vi "UI.vi"(0 "reference in":refnum<class "GUI Alarm Setting.lvclass">, 5 "error in (no error)":errorcluster) -> (14 "reference out":refnum<class "GUI Alarm Setting.lvclass">, 19 "error out":errorcluster)   [LabVIEW 2019, in "GUI Alarm Setting.lvclass"]
uses:
  GUI Alarm Setting.lvclass
  D:/GIT H4000/H4000/src/GUI_class/GUI.lvclass
  GUI_class/GUI.lvclass/GUI.ctl
  GUI_class/Set Win State.vi
  GUI_class/protected/GetSheredData.vi
  GUI_class/GUI.lvclass
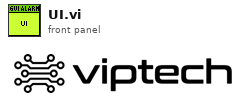
[diagram p1: front panel]
types:
  T1 = enum32{"Invalid", "Standard", "Closed", "Hidden", "Minimized", "Maximized"}
  T2 = enum32{"invalid app kind", "Development System", "Run Time System", "Student Edition", "Embedded LabVIEW", "Evaluation", "Custom"}
  T3 = cluster{"Core":cluster{"Current VI Reference":refnum<vi>, "Close Panel on Exit?":bool}, "file customer":string, "file developer":string, "valid data":bool}
  T4 = cluster{"Current VI Reference":refnum<vi>, "Close Panel on Exit?":bool}
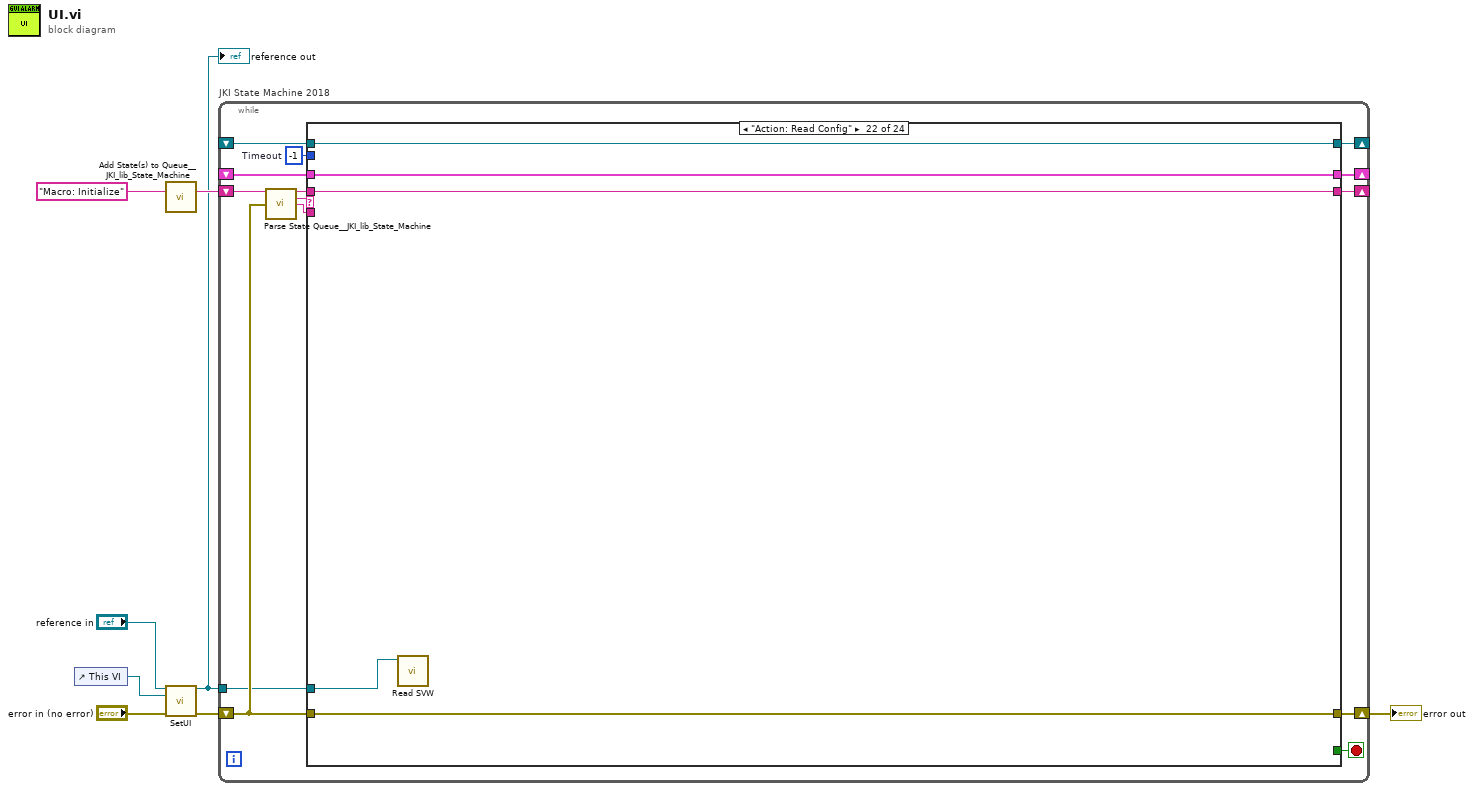
[diagram p0: block diagram]
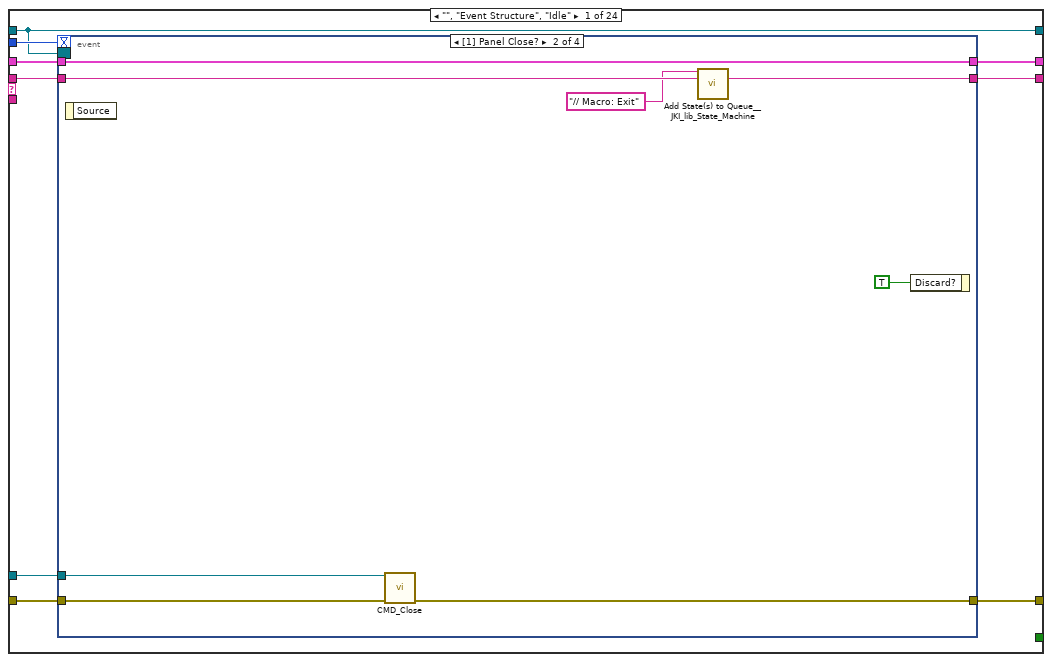
[diagram p2: hidden frame]
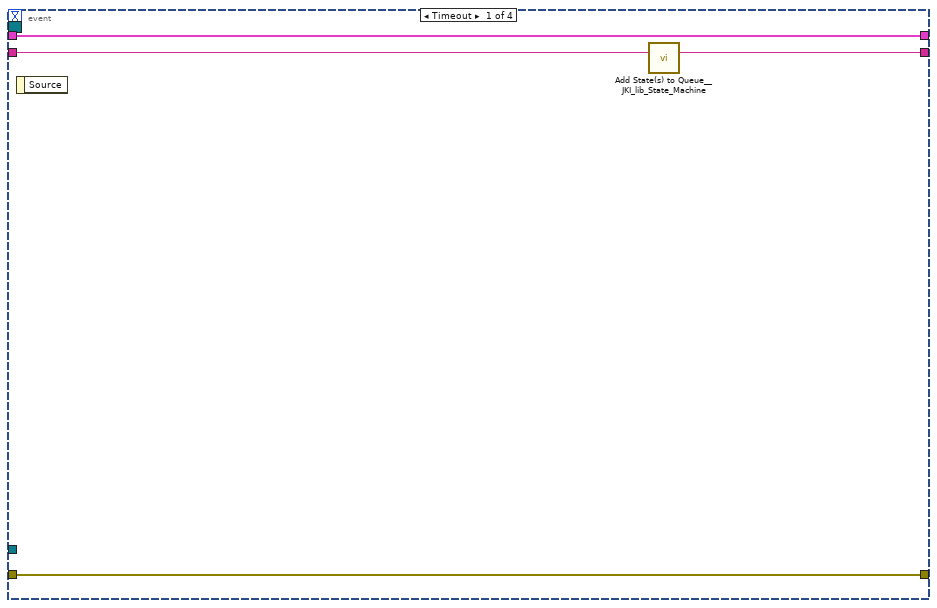
[diagram p3: hidden frame]
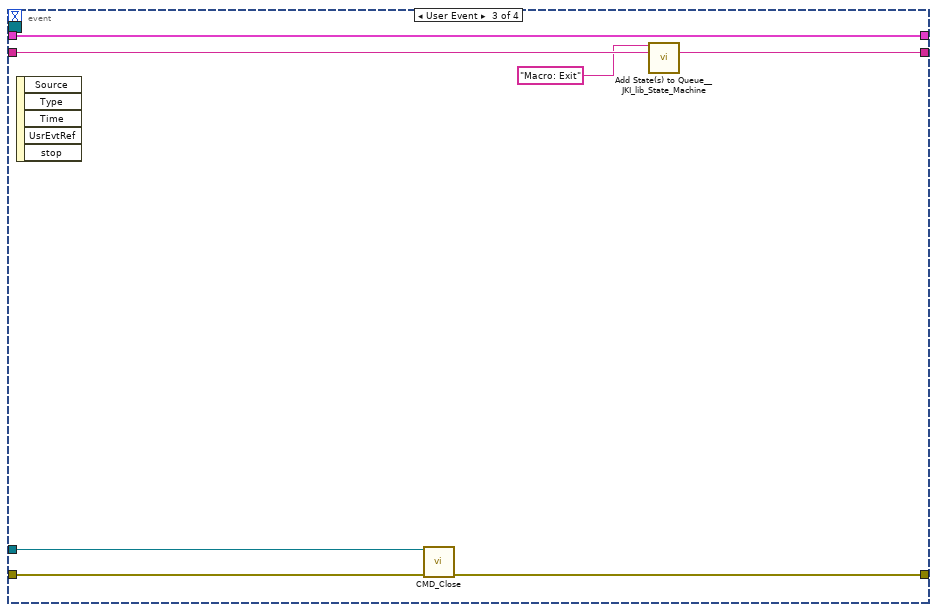
[diagram p4: hidden frame]
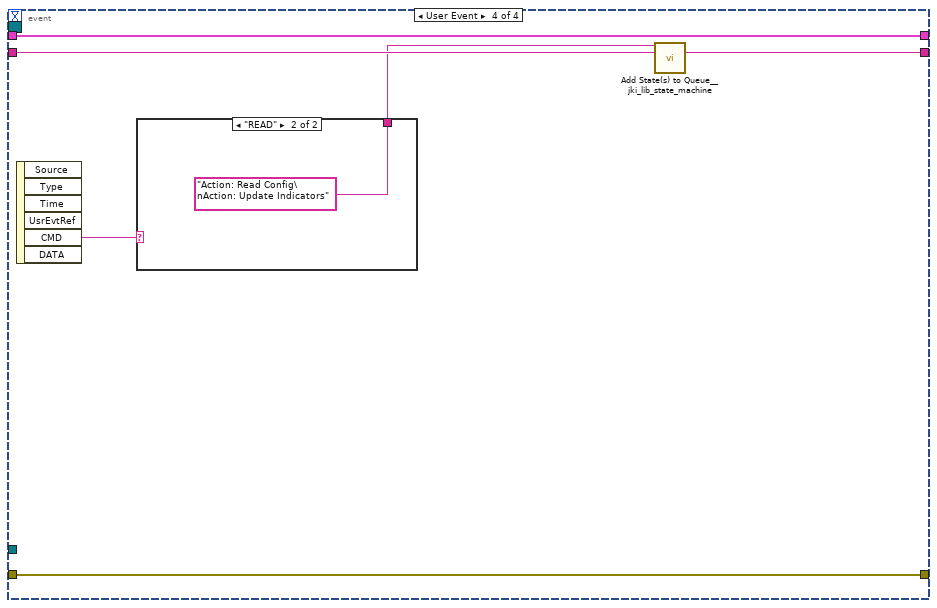
[diagram p5: hidden frame]
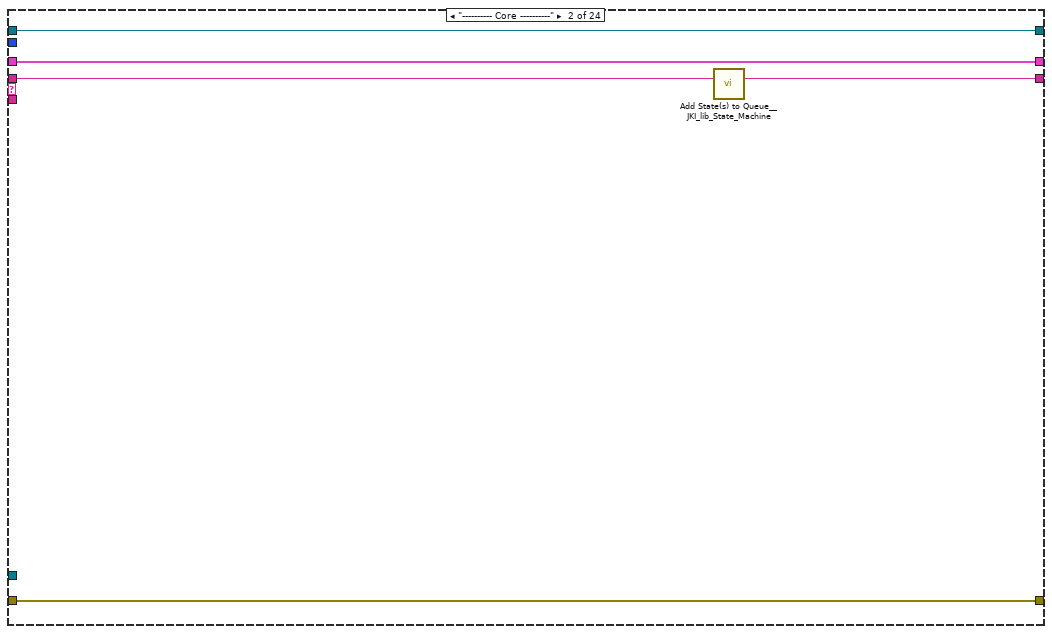
[diagram p7: hidden frame]
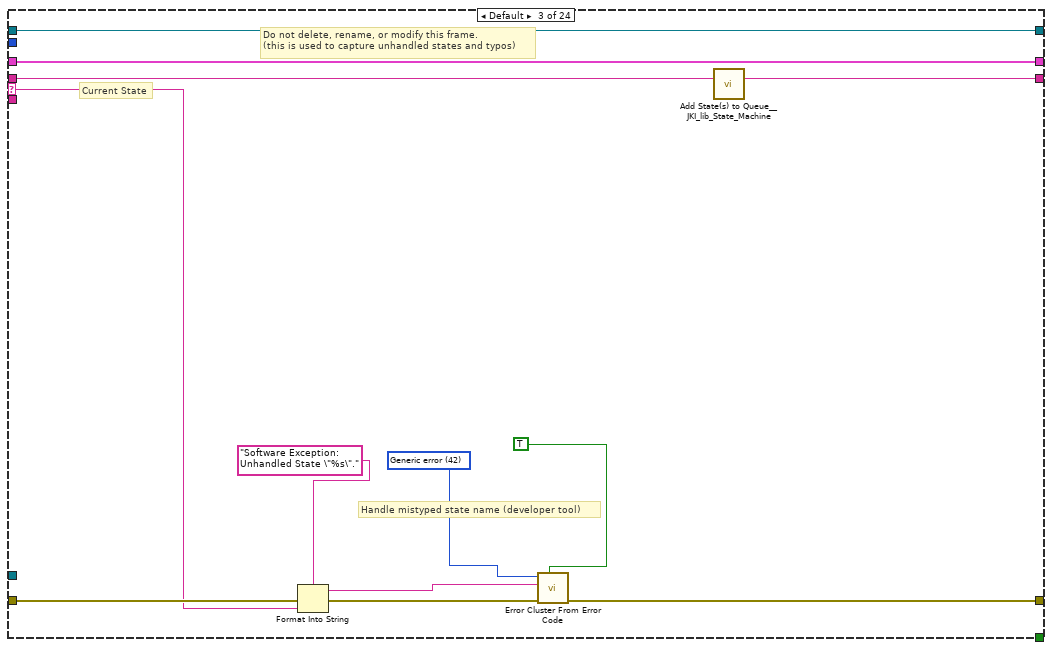
[diagram p8: hidden frame]
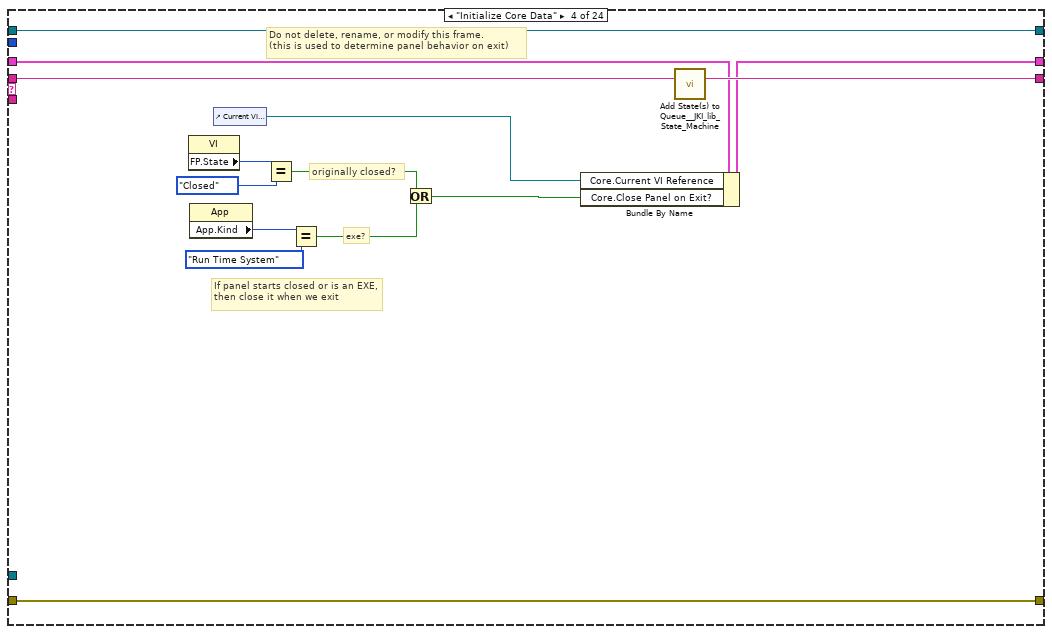
[diagram p9: hidden frame]
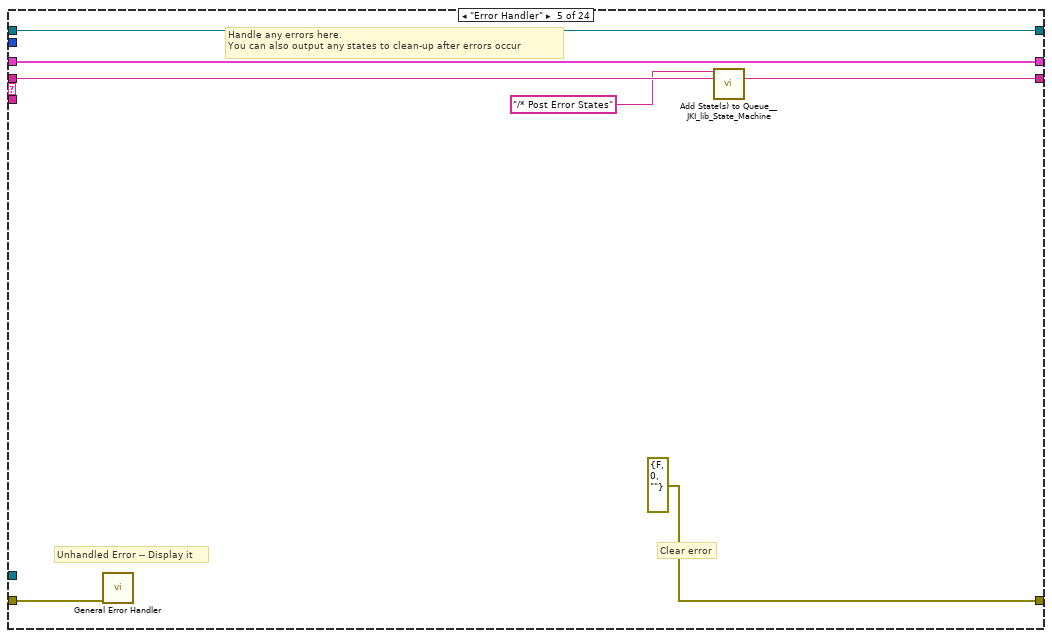
[diagram p10: hidden frame]
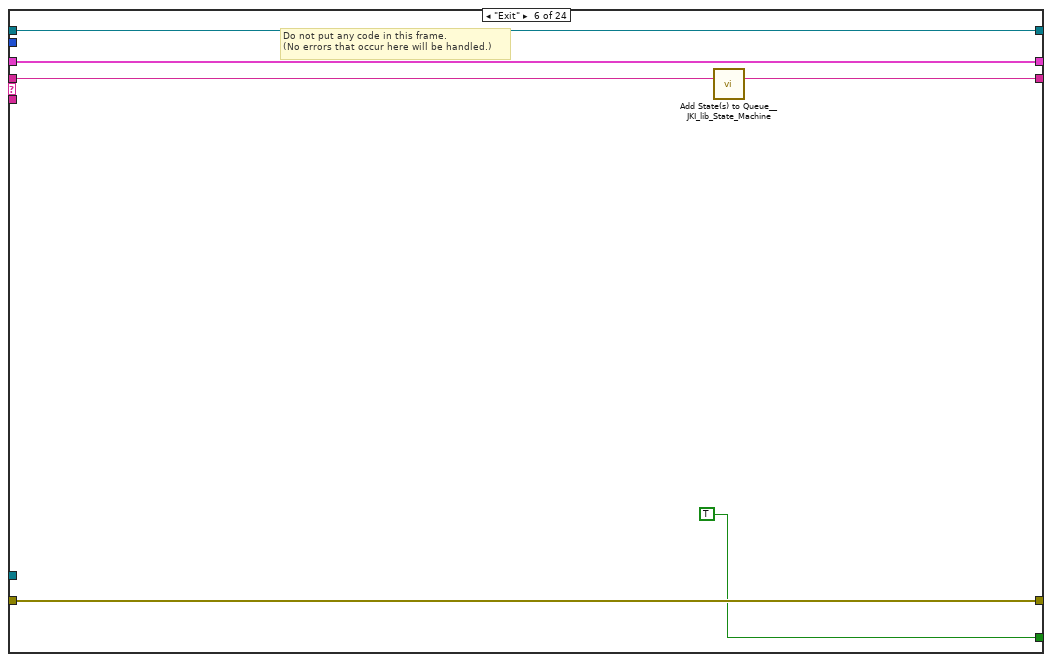
[diagram p11: hidden frame]
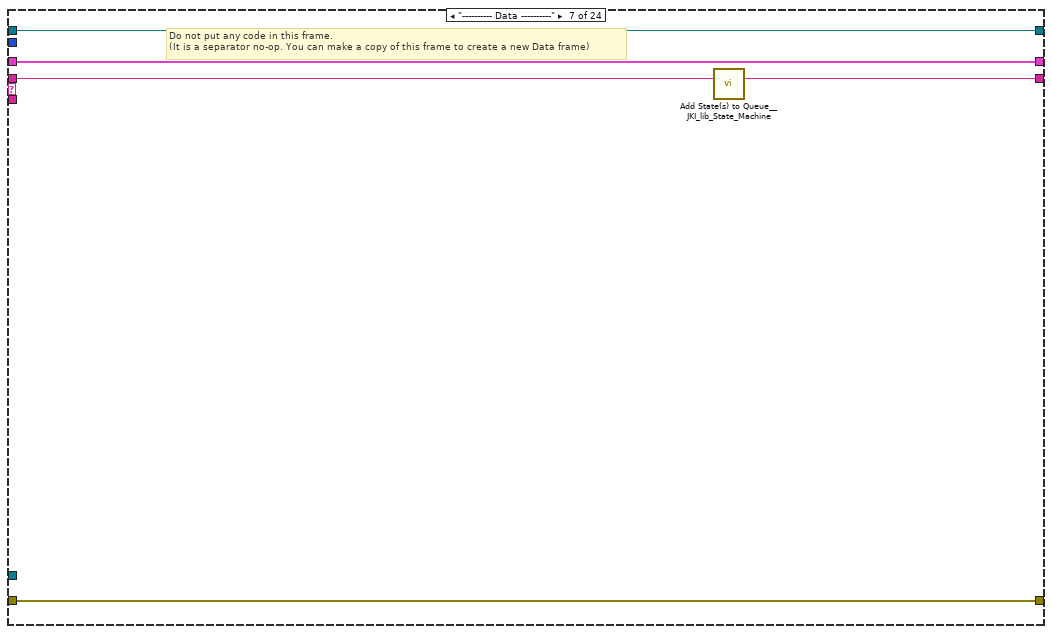
[diagram p12: hidden frame]
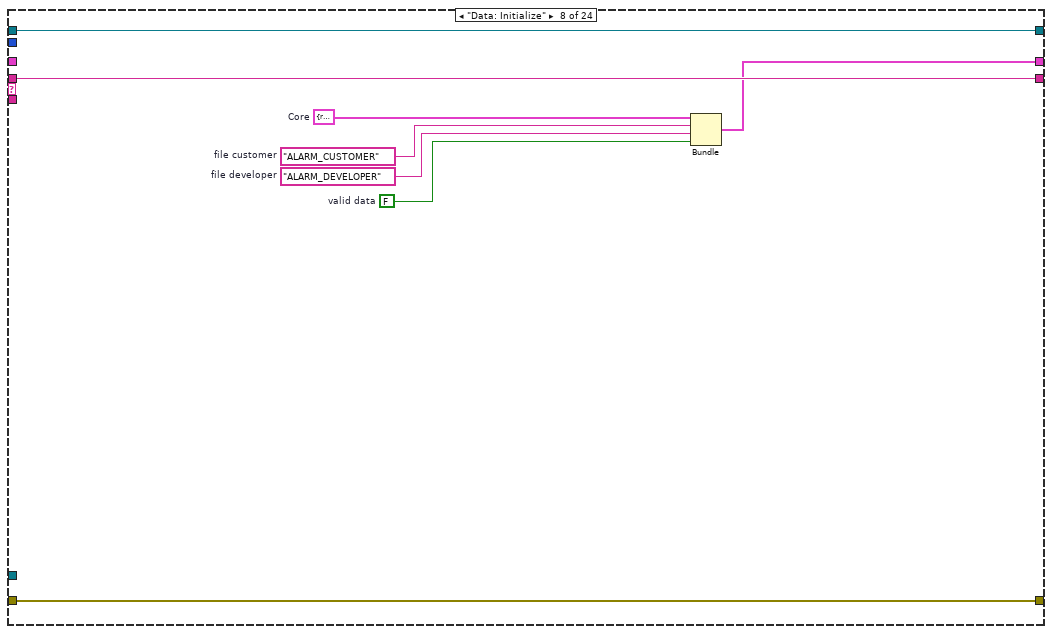
[diagram p13: hidden frame]
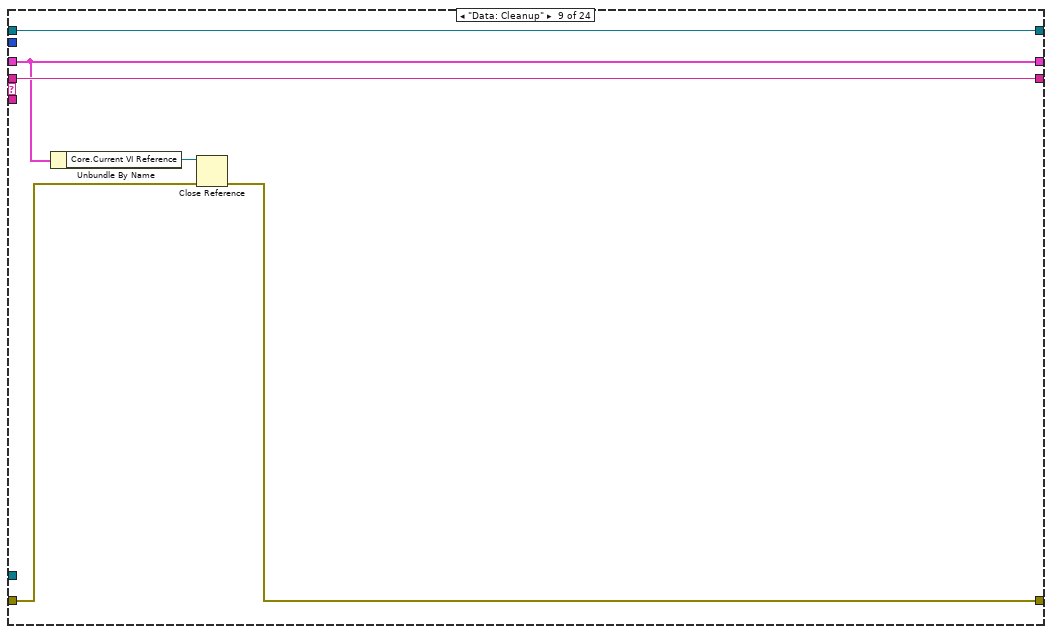
[diagram p14: hidden frame]
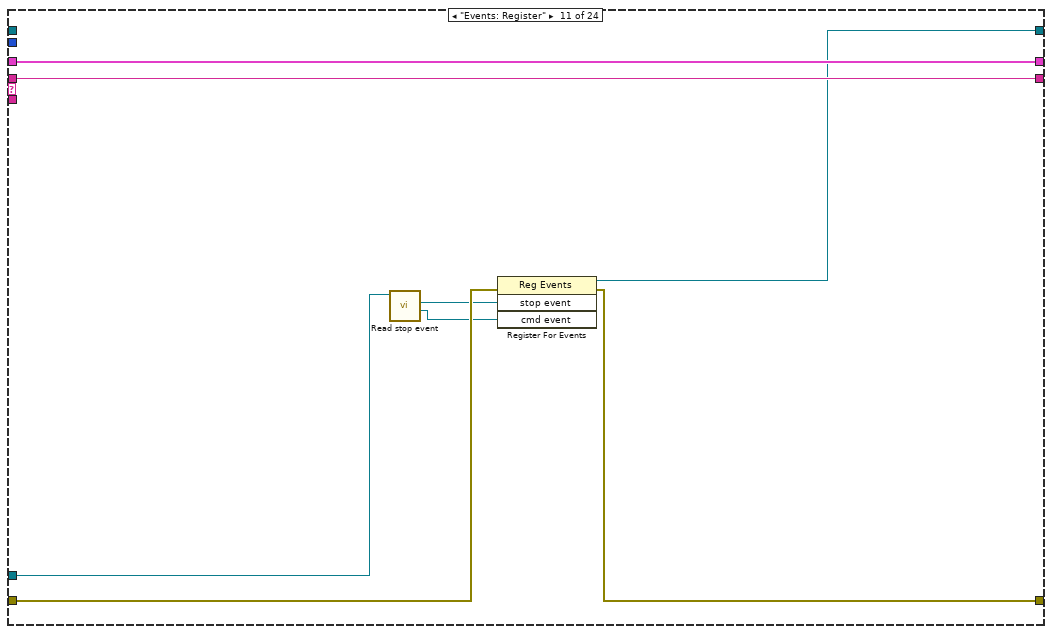
[diagram p16: hidden frame]
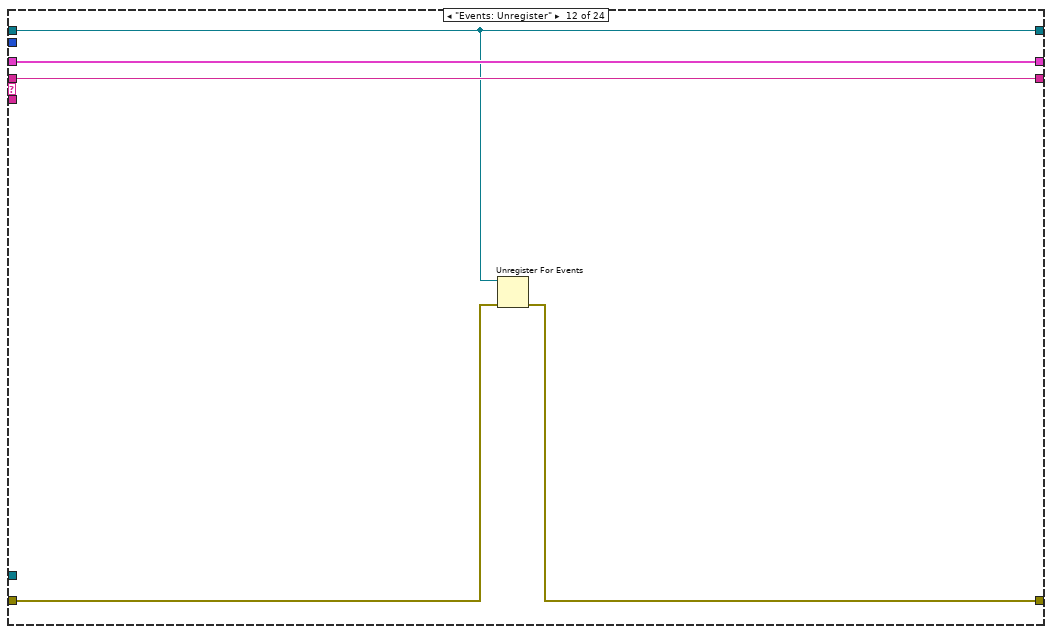
[diagram p17: hidden frame]
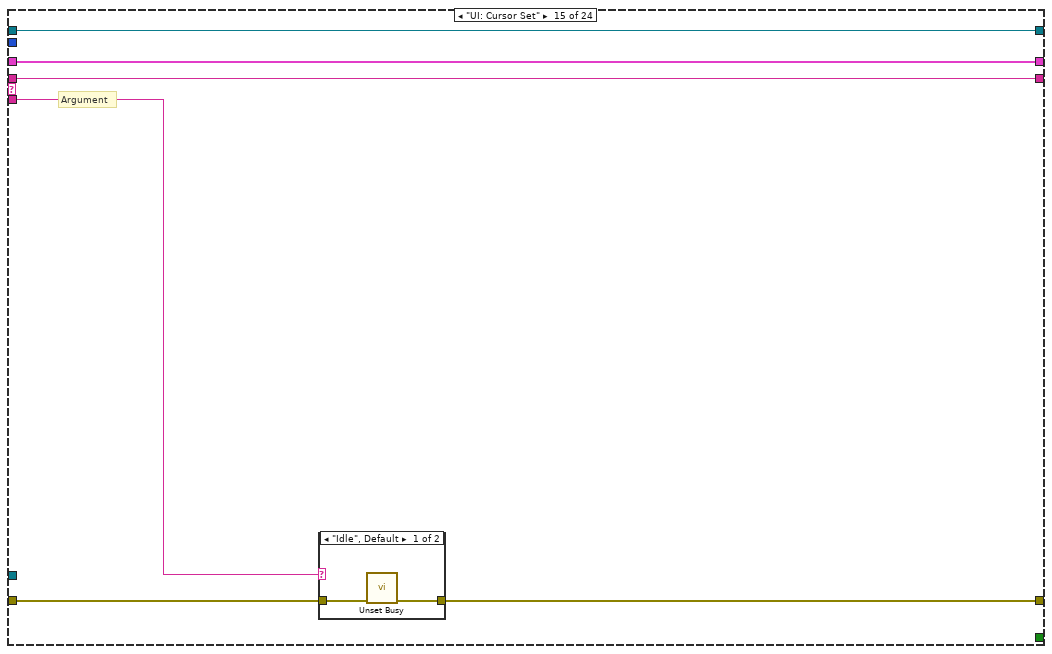
[diagram p20: hidden frame]
diagram:
  n1 = control-ref of="This VI"() -> (w3:refnum<vi>)
  n2 = call <vilib>:"Add State(s) to Queue__JKI_lib_State_Machine.vi"("State(s) in (\"\")"="Macro: Initialize") -> ("States Out"=w8:string)  [unwired: 14 in]
  n3 = call "SetUI.vi"("reference in"="reference in", "UI VI"=w3, "error in (no error)"="error in (no error)") -> ("reference out"=w1:refnum<class "GUI Alarm Setting.lvclass">, "error out"=w2:errorcluster)  [unwired: 11 in]
  "reference out" <- w1
  n4 = while "JKI State Machine 2018" {
    shift-right: [w15] -> _
    shift-left: _ -> [w14]
    shift-right: [w18] -> w6
    shift-left: w2 -> [w12]
    shift-right: [w17] -> _
    shift-left: w8 -> [w19]
    tunnel: w1 -> [w11]
    shift-right: [w10] -> _
    shift-left: _ -> [w9]
    stop <- w16 stop-if-true
    w13 = -1  # Timeout
    n5 = call <vilib>:"Parse State Queue__JKI_lib_State_Machine.vi"("State Queue"=w19, "Error In (no error)"=w12) -> ("Remaining States"=w21:string, "Current State"=w22:string, "Arguments"=w20:string)  [unwired: 11 in]
    n6 = case shown="\"Action: Read Config\"" w22 {
      selector: w22 -> [_ _ w64 _ _ _ _ _ _ _ _ _ _ _ _ _ _ _ _ _ _ _ _ _]
      tunnel: w21 -> [w31 w62 w68 w88 w95 w101 w106 w114 w120 w124 w132 w137 w141 w145 w151 w162 w231 w237 w243 w255 w259 w263 w268 w272]
      tunnel: w20 -> [_ _ _ _ _ _ _ _ _ _ _ _ _ _ w147 w157 _ _ _ _ _ _ _ _]
      tunnel: w14 -> [w29 w59 w66 w81 w92 w99 w103 _ w116 w122 w131 w136 w139 w144 w150 w159 w229 w234 w240 w252 w257 w260 w266 w269]
      tunnel: [w28 w60 w70 w85 errorcluster {"status"=FALSE, "code"=0, "source"=""} ("error out") w98 w104 w112 w117 w123 w129 w133 w140 w143 w148 w160 w230 w235 w241 w253 w258 w261 w265 w270] -> w18
      tunnel: w12 -> [w27 w60 w69 w85 w91 w98 w104 w112 w118 w123 w128 w134 w140 w143 w149 w161 w230 w235 w241 w253 w258 w261 w265 w270]
      tunnel: [w30 w61 w67 w87 w94 w100 w105 w114 w120 w124 w132 w137 w141 w145 w151 w162 w231 w236 w242 w254 w259 w263 w268 w272] -> w17
      tunnel: [_ _ _ _ _ TRUE _ _ _ _ _ _ _ _ _ _ _ _ _ _ _ _ _ _] -> w16
      tunnel: [w26 w59 w66 w86 w92 w99 w103 w113 w116 w122 w131 w136 w139 w144 w150 w159 w229 w234 w240 w252 w257 w260 w266 w269] -> w15
      tunnel: w13 -> [w25 _ _ _ _ _ _ _ _ _ _ _ _ _ _ _ _ _ _ _ _ _ _ _]
      tunnel: w11 -> [w24 _ _ _ _ _ _ _ _ _ w127 _ _ _ _ _ _ _ _ _ _ w262 _ _]
      tunnel: [w23 w58 w63 w75 w89 w96 w102 w110 w115 w121 w130 w135 w138 w142 w146 w156 w228 w232 w238 w245 w256 w264 w267 w271] -> w10
      tunnel: w9 -> [w23 w58 w63 w75 w89 w96 w102 w110 w115 w121 _ w135 w138 w142 w146 w156 w228 w232 w238 w245 w256 w264 w267 w271]
      frame "", "Event Structure", "Idle" {
        n7 = event shown="[1] Panel Close?" {
          selector: w23 -> [_ _ _ _]
          dyn-events: _ -> [_ _ _ _]
          timeout: w25 -> [_ _ _ _]
          tunnel: w31 -> [w35 w43 w50 w52]
          tunnel: [w34 w42 w49 w53] -> w30
          tunnel: w29 -> [w32 w41 w48 w55]
          tunnel: [w33 w36 w44 w56] -> w28
          tunnel: w27 -> [w33 w37 w45 w56]
          tunnel: [w32 w41 w48 w55] -> w26
          tunnel: w24 -> [_ w38 w46 _]
          event Timeout {
            n8 = event-data() -> ()  [unwired: 1 in, 1 out]
            n9 = call <vilib>:"Add State(s) to Queue__JKI_lib_State_Machine.vi"("State(s) in (\"\")"=w35) -> ("States Out"=w34:string)  [unwired: 14 in]
          }
          event Panel Close? {
            n10 = event-data() -> ()  [unwired: 1 in, 1 out]
            n11 = call "CMD_Close.vi"("reference in"=w38, "error in (no error)"=w37) -> ("error out"=w36:errorcluster)  [unwired: 12 in, 1 out]
            n12 = call <vilib>:"Add State(s) to Queue__JKI_lib_State_Machine.vi"("State(s) in Front (\"\")"="// Macro: Exit", "State(s) in (\"\")"=w43) -> ("States Out"=w42:string)  [unwired: 13 in]
            n13 = event-data("Discard?"=TRUE) -> ()  [unwired: 1 in, 1 out]
          }
          event User Event {
            n14 = event-data() -> ()  [unwired: 1 in, 5 out]
            n15 = call "CMD_Close.vi"("reference in"=w46, "error in (no error)"=w45) -> ("error out"=w44:errorcluster)  [unwired: 12 in, 1 out]
            n16 = call <vilib>:"Add State(s) to Queue__JKI_lib_State_Machine.vi"("State(s) in Front (\"\")"="Macro: Exit", "State(s) in (\"\")"=w50) -> ("States Out"=w49:string)  [unwired: 13 in]
          }
          event User Event {
            n17 = event-data() -> ("CMD"=w54:string)  [unwired: 1 in, 5 out]
            n18 = case shown="\"READ\"" w54 {
              tunnel: [_ "Action: Read Config\nAction: Update Indicators" ("State(s) in Front (\"\")")] -> w51
              frame "False", Default {
              }
              frame "READ" {
              }
            }
            n19 = call <vilib>:"Add State(s) to Queue__jki_lib_state_machine.vi"("State(s) in Front (\"\")"=w51, "State(s) in (\"\")"=w52) -> ("States Out"=w53:string)  [unwired: 13 in]
          }
        }
      }
      frame "---------- Core ----------" {
        n20 = call <vilib>:"Add State(s) to Queue__JKI_lib_State_Machine.vi"("State(s) in (\"\")"=w62) -> ("States Out"=w61:string)  [unwired: 14 in]
      }
      frame Default {
        w73 = 42 items=["No error", "Argument error", "Memory is full", "Out of zone", "End of file", "File already open", "Generic file I/O error", "File not found", "File permission error", "Disk is full", "Duplicate path", "Too many files open", "System feature not enabled", "Resource file not found", "Cannot add resource", "Resource not found", "Image not found", "Image memory error", "Pen does not exist", "Config type invalid", "Config token not found", "Config parse error", "Config memory error", "Bad external code format", "Bad external code offset", "External code not present", "Null window", "Destroy window error", "Null menu", "Print aborted", "Bad print record", "Print driver error", "Windows error during printing", "Memory error during printing", "Print dialog error", "Generic print error", "Invalid device refnum", "Device not found", "Device parameter error", "Device unit error", "Cannot open device", "Device call aborted", "Generic error", "Cancelled by user", "Object ID too low", "Object ID too high", "Object not in heap", "Unknown heap", "Unknown object (invalid DefProc)", "Unknown object (DefProc not in table)", "Message out of range", "Invalid (null) method", "Unknown message", "Manager call not supported", "Bad address", "Network operation in progress", "Network operation timed out", "Connection is busy", "Network attribute not supported", "Network error", "Address in use", "System out of memory", "Connection aborted", "Connection refused", "Not connected", "Already connected", "Connection closed", "Initialization error (interapplication manager)", "Bad occurrence", "Wait on unbound occurrence handler", "Occurrence queue overflow", "Datalog type conflict", "Unused", "Unrecognized type (interapplication manager)", "Memory corrupt", "Failed to make temporary DLL", "Old CIN version", "Drag socket not found", "Failed to load drop-object", "Failed to register OLE object", "Failed to release OLE object", "Format specifier type mismatch", "Unknown format specifier", "Too few format specifiers", "Too many format specifiers", "Scan failed", "Newer CIN version", "Error converting to variant", "Runtime menu error", "Password tampered", "Variant attribute not found", "Incompatible variant data type", "Event data is not available", "Event Store is not present", "Occurrence is not found", "Event Queue is not created", "Event info is not available", "Refnum passed is NULL", "Error retrieving Class GUID", "Error retrieving CoClass GUID", "Error retrieving TypeLib GUID.", "Bad built application magic bytes.", "Specific driver is different from the specific driver associated with the Logical Name.", "There is no session opened to the class driver.", "Max Error", "MAX - Error with config objects", "MAX - Error loading configuration", "MAX - Group not supported"]
        # "Current State"
        # "Do not delete, rename, or modify this frame.\n(this is used to capture unhandled states and typos)"
        # "Handle mistyped state name (developer tool)"
        n21 = Format Into String(format string="Software Exception: Unhandled State \"%s\"." ("message"), error in=w69, w64) -> (resulting string=w72:string, error out=w71:errorcluster)  [unwired: 1 in]
        n22 = call <vilib>:"Error Cluster From Error Code.vi"("show call chain? (False)"=TRUE, "error in (no error)"=w71, "error message (\"\")"=w72, "error code (0)"=w73) -> ("error out"=w70:errorcluster)  [unwired: 5 in]
        n23 = call <vilib>:"Add State(s) to Queue__JKI_lib_State_Machine.vi"("State(s) in (\"\")"=w68) -> ("States Out"=w67:string)  [unwired: 14 in]
      }
      frame "Initialize Core Data" {
        # "Do not delete, rename, or modify this frame.\n(this is used to determine panel behavior on exit)"
        # "originally closed?"
        # "exe?"
        # "If panel starts closed or is an EXE, then close it when we exit"
        n24 = property class="VI"() -> ("FP.State"=w78:T1)  [unwired: 2 in, 2 out]
        n25 = property class="App"() -> ("App.Kind"=w84:T2)  [unwired: 2 in, 2 out]
        n26 = control-ref of="Current VI Reference"() -> (w79:refnum<vi>)
        n27 = Equal?(x=w78, y=T1."Closed" ("Front Panel Window:State")) -> (x = y?=w76:bool)
        n28 = Equal?(x=w84, y=T2."Run Time System" ("Application:Kind")) -> (x = y?=w82:bool)
        n29 = Or(x=w76, y=w82) -> (x .or. y?=w80:bool)
        n30 = Bundle By Name(cluster=w81, "Core.Current VI Reference"=w79, "Core.Close Panel on Exit?"=w80) -> (w86:T3)
        n31 = call <vilib>:"Add State(s) to Queue__JKI_lib_State_Machine.vi"("State(s) in (\"\")"=w88) -> ("States Out"=w87:string)  [unwired: 14 in]
      }
      frame "Error Handler" {
        # "Unhandled Error -- Display it"
        # "Handle any errors here.\nYou can also output any states to clean-up after errors occur"
        # "Clear error"
        n32 = call <vilib>:"General Error Handler.vi"("error in (no error)"=w91) -> ()  [unwired: 10 in, 5 out]
        n33 = call <vilib>:"Add State(s) to Queue__JKI_lib_State_Machine.vi"("State(s) in Front (\"\")"="/* Post Error States", "State(s) in (\"\")"=w95) -> ("States Out"=w94:string)  [unwired: 13 in]
      }
      frame "Exit" {
        # "Do not put any code in this frame.\n(No errors that occur here will be handled.)"
        n34 = call <vilib>:"Add State(s) to Queue__JKI_lib_State_Machine.vi"("State(s) in (\"\")"=w101) -> ("States Out"=w100:string)  [unwired: 14 in]
      }
      frame "---------- Data ----------" {
        # "Do not put any code in this frame.\n(It is a separator no-op. You can make a copy of this frame to create a new Data frame)"
        n35 = call <vilib>:"Add State(s) to Queue__JKI_lib_State_Machine.vi"("State(s) in (\"\")"=w106) -> ("States Out"=w105:string)  [unwired: 14 in]
      }
      frame "Data: Initialize" {
        w107 = FALSE  # valid data
        w108 = "ALARM_DEVELOPER"  # file developer
        w109 = "ALARM_CUSTOMER"  # file customer
        w111 = T4 {"Current VI Reference"=refnum, "Close Panel on Exit?"=FALSE}  # Core
        n36 = Bundle("Core"=w111, "file customer"=w109, "file developer"=w108, "valid data"=w107) -> (w113:T3)  [unwired: 1 in]
      }
      frame "Data: Cleanup" {
        n37 = Unbundle By Name(w116) -> ("Core.Current VI Reference"=w119:refnum<vi>)
        n38 = Close Reference(reference=w119, error in (no error)=w118) -> (error out=w117:errorcluster)
      }
      frame "---------- Events ----------" {
      }
      frame "Events: Register" {
        n39 = call "Read stop event.vi"("GUI in"=w127) -> ("cmd event"=w125:refnum<user-event>, "stop event"=w126:refnum<user-event>)  [unwired: 8 in, 1 out]
        n40 = register-events(error in=w128, w126, w125) -> (reference out=w130:refnum<event-registration>, error out=w129:errorcluster)  [unwired: 1 in]
      }
      frame "Events: Unregister" {
        n41 = Unregister For Events(event registration refnum=w135, error in=w134) -> (error out=w133:errorcluster)
      }
      frame "---------- UI ----------" {
      }
      frame "UI: Initialize" {
      }
      frame "UI: Cursor Set" {
        # "Argument"
        n42 = case shown="\"Idle\", Default" w147 {
          tunnel: w149 -> [w153 w155]
          tunnel: [w152 w154] -> w148
          frame "Idle", Default {
            n43 = call <vilib>:"Unset Busy.vi"("error in (no error)"=w153) -> ("error out"=w152:errorcluster)  [unwired: 10 in]
          }
          frame "Busy" {
            n44 = call <vilib>:"Set Busy.vi"("error in (no error)"=w155) -> ("error out"=w154:errorcluster)  [unwired: 9 in, 1 out]
          }
        }
      }
      frame "UI: Front Panel State" {
        # "Argument"
        n45 = Unbundle By Name(w159) -> ("Core.Current VI Reference"=w158:refnum<vi>)
        n46 = case shown="\"Minimize\", \"Minimized\"" w157 {
          tunnel: w161 -> [w168 w183 w194 w207 w220]
          tunnel: [w170 w184 w196 w209 w222] -> w160
          tunnel: w158 -> [w169 w181 w195 w208 w221]
          frame "Open", "Standard", Default {
            w163 = T1."Standard" ("State")
            n47 = property class="VI"(reference=w169, error in=w168) -> (reference out=w166:refnum<vi>, error out=w167:errorcluster, "FP.State"=w165:T1)
            n48 = Not Equal?(x=w165, y=w163) -> (x != y?=w164:bool)
            n49 = case shown="True" w164 {
              tunnel: [w174 w176] -> w170
              tunnel: w167 -> [w173 w176]
              tunnel: w166 -> [w172 _]
              tunnel: w163 -> [w171 _]
              frame True {
                n50 = invoke class="VI" method="FP.Open"(reference=w172, error in=w173, "Activate"=TRUE, "State"=w171) -> (error out=w174:errorcluster)  [unwired: 1 in, 4 out]
              }
              frame False {
              }
            }
          }
          frame "Close", "Closed" {
            n51 = property class="VI"(reference=w181, error in=w183) -> (reference out=w180:refnum<vi>, error out=w182:errorcluster, "FP.State"=w178:T1)
            n52 = Not Equal?(x=w178, y=T1."Closed" ("Front Panel Window:State")) -> (x != y?=w177:bool)
            n53 = case shown="True" w177 {
              tunnel: [w185 w188] -> w184
              tunnel: w182 -> [w185 w187]
              tunnel: w180 -> [_ w186]
              frame False {
              }
              frame True {
                n54 = invoke class="VI" method="FP.Close"(reference=w186, error in=w187) -> (error out=w188:errorcluster)  [unwired: 1 in, 2 out]
              }
            }
          }
          frame "Hidden", "Hide" {
            w189 = T1."Hidden" ("State")
            n55 = property class="VI"(reference=w195, error in=w194) -> (reference out=w192:refnum<vi>, error out=w193:errorcluster, "FP.State"=w191:T1)
            n56 = Not Equal?(x=w191, y=w189) -> (x != y?=w190:bool)
            n57 = case shown="True" w190 {
              tunnel: [w200 w201] -> w196
              tunnel: w193 -> [w199 w201]
              tunnel: w192 -> [w198 _]
              tunnel: w189 -> [w197 _]
              frame True {
                n58 = invoke class="VI" method="FP.Open"(reference=w198, error in=w199, "State"=w197) -> (error out=w200:errorcluster)  [unwired: 2 in, 4 out]
              }
              frame False {
              }
            }
          }
          frame "Minimize", "Minimized" {
            w202 = T1."Minimized" ("State")
            n59 = property class="VI"(reference=w208, error in=w207) -> (reference out=w205:refnum<vi>, error out=w206:errorcluster, "FP.State"=w204:T1)
            n60 = Not Equal?(x=w204, y=w202) -> (x != y?=w203:bool)
            n61 = case shown="True" w203 {
              tunnel: [w213 w214] -> w209
              tunnel: w206 -> [w212 w214]
              tunnel: w205 -> [w211 _]
              tunnel: w202 -> [w210 _]
              frame True {
                n62 = invoke class="VI" method="FP.Open"(reference=w211, error in=w212, "State"=w210) -> (error out=w213:errorcluster)  [unwired: 2 in, 4 out]
              }
              frame False {
              }
            }
          }
          frame "Maximize", "Maximized" {
            w215 = T1."Maximized" ("State")
            n63 = property class="VI"(reference=w221, error in=w220) -> (reference out=w218:refnum<vi>, error out=w219:errorcluster, "FP.State"=w217:T1)
            n64 = Not Equal?(x=w217, y=w215) -> (x != y?=w216:bool)
            n65 = case shown="True" w216 {
              tunnel: [w226 w227] -> w222
              tunnel: w219 -> [w225 w227]
              tunnel: w218 -> [w224 _]
              tunnel: w215 -> [w223 _]
              frame True {
                n66 = invoke class="VI" method="FP.Open"(reference=w224, error in=w225, "State"=w223) -> (error out=w226:errorcluster)  [unwired: 2 in, 4 out]
              }
              frame False {
              }
            }
          }
        }
      }
      frame "---------- Macro ----------" {
      }
      frame "Macro: Initialize" {
        n67 = call <vilib>:"Add State(s) to Queue__JKI_lib_State_Machine.vi"("State(s) in Front (\"\")"="Data: Initialize\nInitialize Core Data\nEvents: Register\nUI: Initialize\n", "State(s) in (\"\")"=w237) -> ("States Out"=w236:string)  [unwired: 13 in]
      }
      frame "Macro: Update" {
        n68 = call <vilib>:"Add State(s) to Queue__JKI_lib_State_Machine.vi"("State(s) in Front (\"\")"="Action: Update Indicators\nAction: Write Config", "State(s) in (\"\")"=w243) -> ("States Out"=w242:string)  [unwired: 13 in]
      }
      frame "Macro: Exit" {
        # "Exit Macro\n(This is called once, when the VI exits)"
        n69 = Unbundle By Name(w252) -> ("Core.Close Panel on Exit?"=w251:bool)
        n70 = Select(t="UI: Front Panel State >> Close", s=w251, f="") -> (s? t:f=w248:string)
        n71 = call <vilib>:"Add State(s) to Queue__JKI_lib_State_Machine.vi"("State(s) in Front (\"\")"="Action: Write Config", "State(s) in (\"\")"=w248, "State(s) at Back (\"\")"="Data: Cleanup\nEvents: Unregister\nExit") -> ("States Out"=w246:string)  [unwired: 12 in]
        n72 = call <vilib>:"Add State(s) to Queue__JKI_lib_State_Machine.vi"("State(s) in Front (\"\")"=w246, "State(s) in (\"\")"=w255) -> ("States Out"=w254:string)  [unwired: 13 in]
      }
      frame "---------- Action ----------" {
      }
      frame "Action: Read Config" {
        n73 = call "Read SVW.vi"("GUI in"=w262) -> ()  [unwired: 10 in, 1 out]
      }
      frame "Action: Write Config" {
      }
      frame "Action: Update Indicators" {
      }
    }
  }
  "error out" <- w6
